vi "ingest.dataflash.vi"(8 "error in":errorcluster, 11 "DataflashIngestStaging in":refnum<class "DataflashIngestStaging.lvclass">) -> (0 "error out":errorcluster, 3 "DataflashIngestStaging out":refnum<class "DataflashIngestStaging.lvclass">)   [LabVIEW 2020, in "DataflashIngestStaging.lvclass"]
doc: "Ingests an ArduPilot DataFlash log file into an existing dataset."
uses:
  DataflashIngestStaging.lvclass
  DataflashIngestStaging.lvclass/DataflashIngestStaging.ctl
  client.lvlib
panel:
  out "out_job out":i32
  in  "staging":i32
  in  "file_path":string
  in  "dataset_rid":string
  in  "out_job":i32
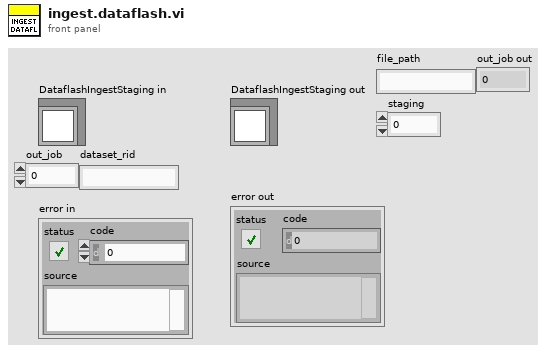
[diagram p1: front panel]
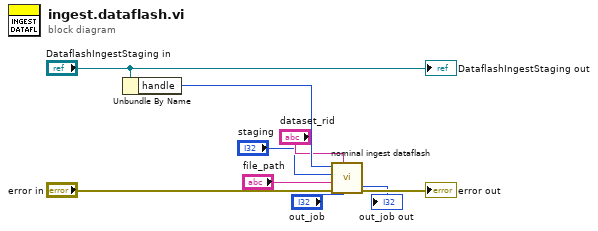
[diagram p0: block diagram]
diagram:
  n1 = Unbundle By Name("DataflashIngestStaging in") -> ("handle"=w7:i32)
  n2 = call "nominal ingest dataflash.vi"("out_job"="out_job", "dataset_rid"="dataset_rid", "error in (no error)"="error in", "file_path"="file_path", "staging"="staging", "client"=w7) -> ("error out"=→"error out":errorcluster, "out_job out"=→"out_job out":i32)  [unwired: 3 in, 1 out]
  "DataflashIngestStaging out" <- "DataflashIngestStaging in"
